vi "Facade.vi"(0 "Data In":T10=[{"Channel Name"=0, "Channel Alias"="", "Remove Channel"=FALSE, "Index"=0}], 2 "Display State In":T6={"Current Channels Info"=[], "Help Prefix"="", "Max Display Size"=8, "Max Size"=0, "Show Buttons"=TRUE, "Data Valid"=refnum, "Show Range"=FALSE, "Range Items"=[], "Range Index"=[]}, 3 "Container State":T9) -> (6 "Data Out":T10, 7 "Display State Out":T6={"Current Channels Info"=[], "Help Prefix"="", "Max Display Size"=8, "Max Size"=0, "Show Buttons"=TRUE, "Data Valid"=refnum, "Show Range"=FALSE, "Range Items"=[], "Range Index"=[]}, 8 "Action":T5)   [LabVIEW 2021, in "myRIO Channel List.xctl"]
uses:
  <vilib>/myRIO/Common/Express VI Framework/xctls/myRIO Channel List/myRIO Channel List.xctl
  <vilib>/myRIO/Common/Express VI Framework/xctls/myRIO Channel List/Data.ctl
  <vilib>/myRIO/Common/Express VI Framework/xctls/myRIO Channel List/typedefs/Channel Data.ctl
  <vilib>/myRIO/Common/Express VI Framework/xctls/myRIO Channel List/typedefs/Remove Channel.ctl
  <vilib>/_xctls/Container State.ctl
  <vilib>/myRIO/Common/Express VI Framework/xctls/myRIO Channel List/State.ctl
  <vilib>/myRIO/Common/Profile Manager Framework/typedefs/Channel Info.ctl
  <vilib>/myRIO/Common/Express VI Framework/typedefs/Data Validate Ref.ctl
  <vilib>/_xctls/Action.ctl
  <vilib>/myRIO/Common/Express VI Framework/xctls/myRIO Channel List/typedefs/Channel View.ctl
  <vilib>/myRIO/Common/Express VI Framework/xctls/myRIO Channel List/typedefs/Error Icon.ctl
  <vilib>/myRIO/Common/Express VI Framework/xctls/myRIO Channel List/typedefs/Add Channel.ctl
  <vilib>/myRIO/Common/Express VI Framework/xctls/myRIO Channel List/typedefs/Update State.ctl
  <vilib>/_xctls/XControlSupport.lvlib
panel:
  in  "Add Channel":T1
  in  "Channels":T2[](array[typedef])
  in  "Scrollbar":i32(c297)
  # "Channel:"
  # "Custom channel name:"
  # "Range:"
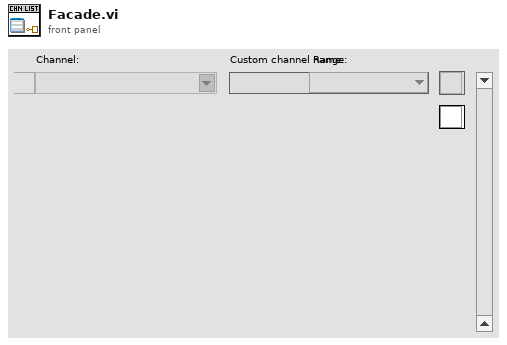
[diagram p1: front panel]
types:
  T1 = typedef "myRIO Channel List.xctl/Add Channel.ctl" = bool
  T2 = typedef "myRIO Channel List.xctl/Channel View.ctl" = cluster{"Error Icon":T3, "Channel Name":string, "Channel Alias":string, "Remove Channel":T4, "Index":i32, "Range":i32}
  T3 = typedef "myRIO Channel List.xctl/Error Icon.ctl" = bool
  T4 = typedef "myRIO Channel List.xctl/Remove Channel.ctl" = bool
  T5 = typedef "XControlSupport.lvlib/Action.ctl" = cluster{"Data Changed?":bool, "State Changed?":bool, "Action Name":string}
  T6 = typedef "myRIO Channel List.xctl/State.ctl" = cluster{"Current Channels Info":T7[], "Help Prefix":string, "Max Display Size":i32, "Max Size":i32, "Show Buttons":bool, "Data Valid":T8, "Show Range":bool, "Range Items":string[], "Range Index":i32[]}
  T7 = typedef "Channel Info.ctl" = cluster{"Channel Name":string, "Alias":string, "Used?":bool, "Not Support?":bool, "Property Bundle":cluster{"Name":string, "Value":variant}[]}
  T8 = typedef "Data Validate Ref.ctl" = refnum<user-event>
  T9 = typedef "XControlSupport.lvlib/Container State.ctl" = cluster{"Indicator?":bool, "Run Mode?":bool, " Refnum":refnum<vi>}
  T10 = typedef "myRIO Channel List.xctl/Data.ctl" = T11[]
  T11 = typedef "myRIO Channel List.xctl/Channel Data.ctl" = cluster{"Channel Name":u16, "Channel Alias":string, "Remove Channel":T4, "Index":i32}
  T12 = typedef "myRIO Channel List.xctl/Update State.ctl" = enum16{"Defer Update", "Allow Update", "Update Channel List", "Update Values", "Update Value", "Update Channel", "Update Index", "Update Scrollbar", "Update Buttons", "Update Container", "Update Help", "Show Or Hide Range"}
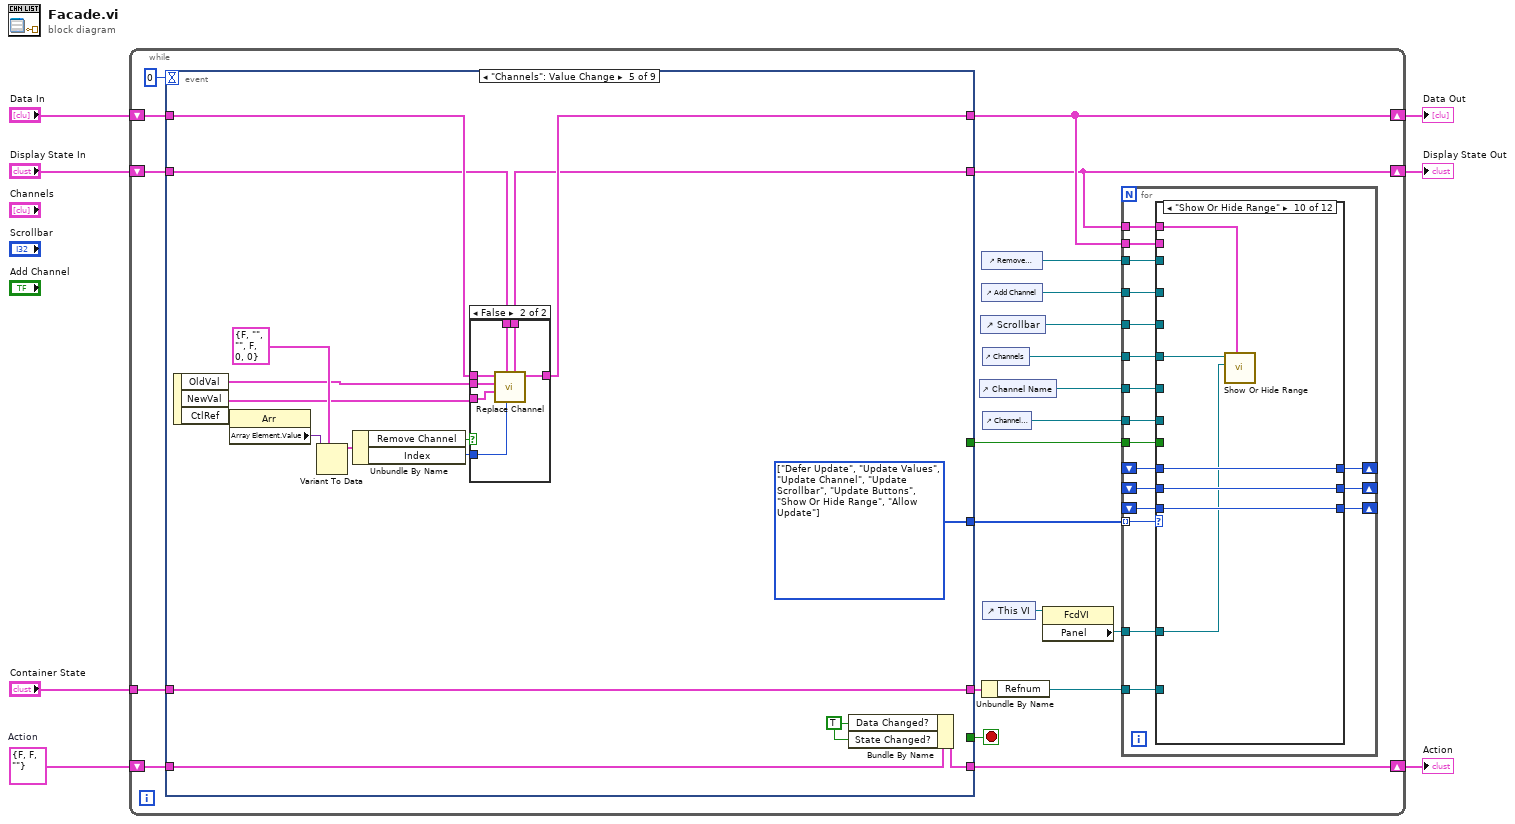
[diagram p0: block diagram]
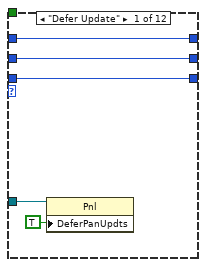
[diagram p2: hidden frame]
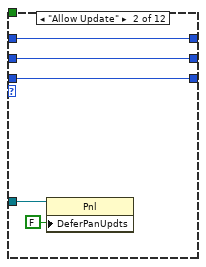
[diagram p3: hidden frame]
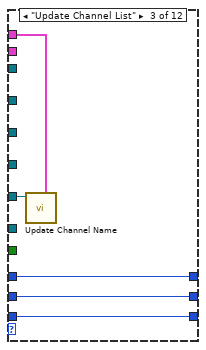
[diagram p4: hidden frame]
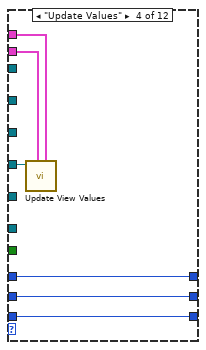
[diagram p5: hidden frame]
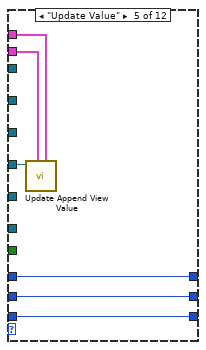
[diagram p6: hidden frame]
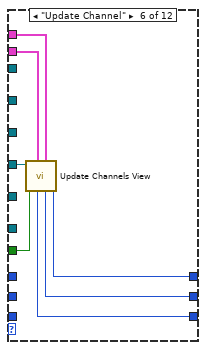
[diagram p7: hidden frame]
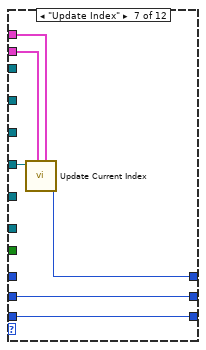
[diagram p8: hidden frame]
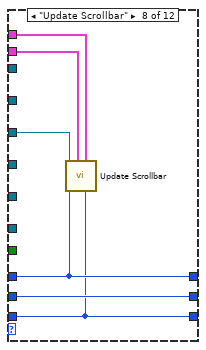
[diagram p9: hidden frame]
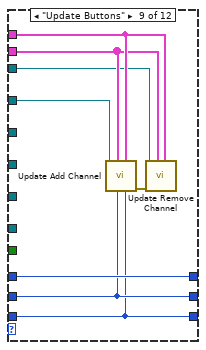
[diagram p10: hidden frame]
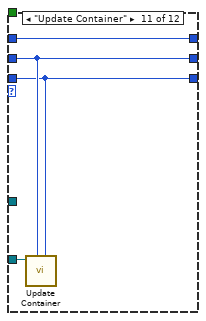
[diagram p11: hidden frame]
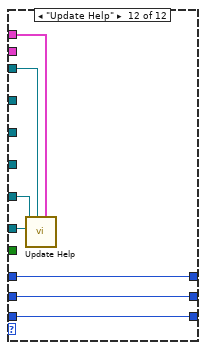
[diagram p12: hidden frame]
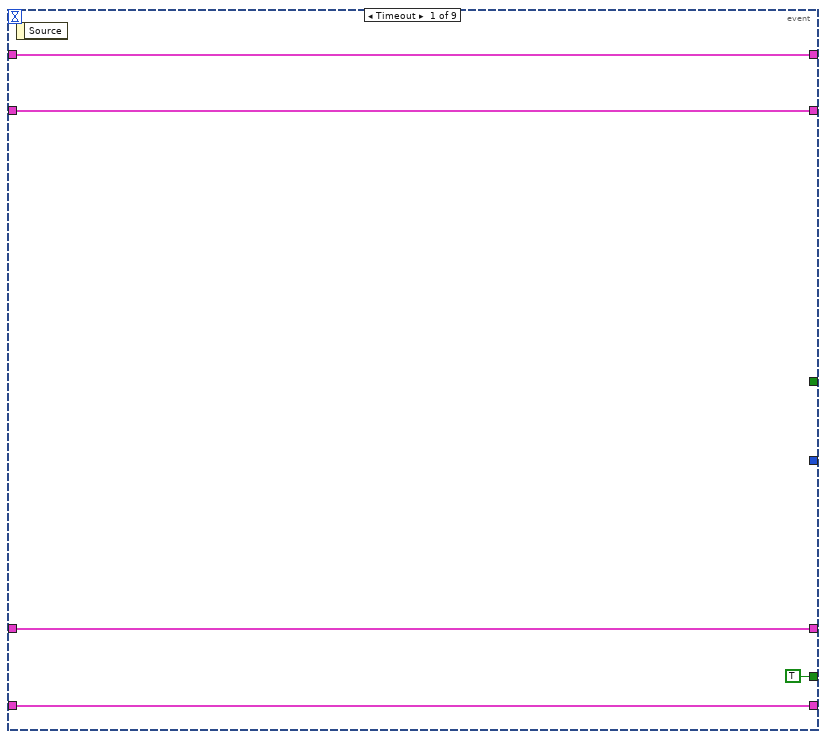
[diagram p13: hidden frame]
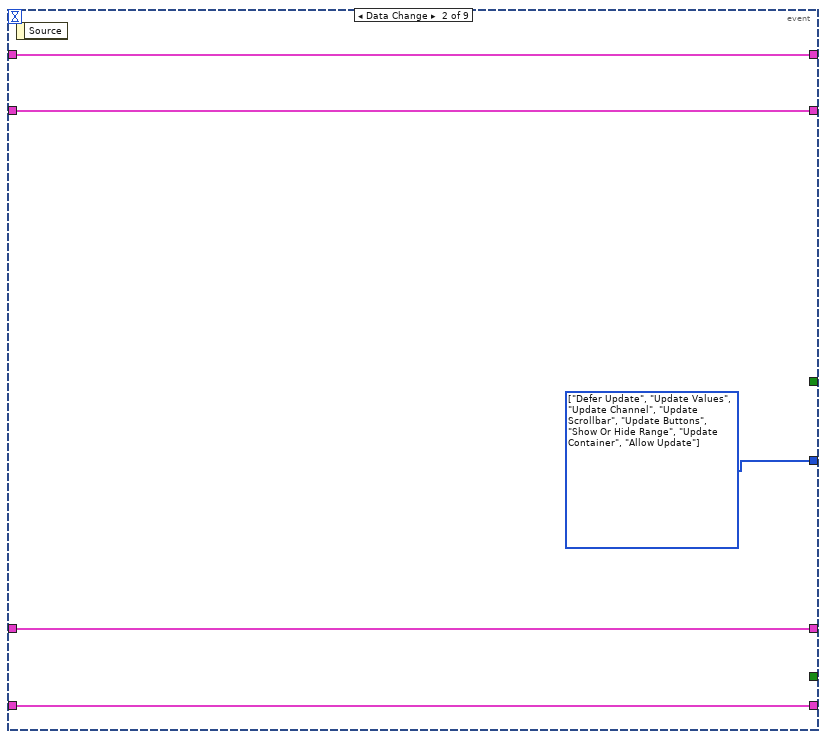
[diagram p14: hidden frame]
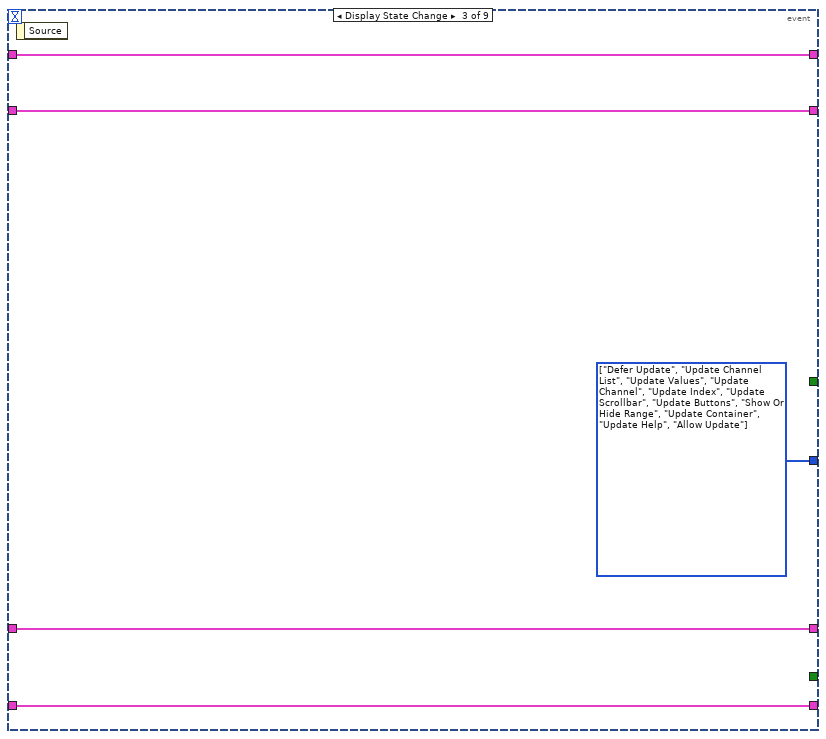
[diagram p15: hidden frame]
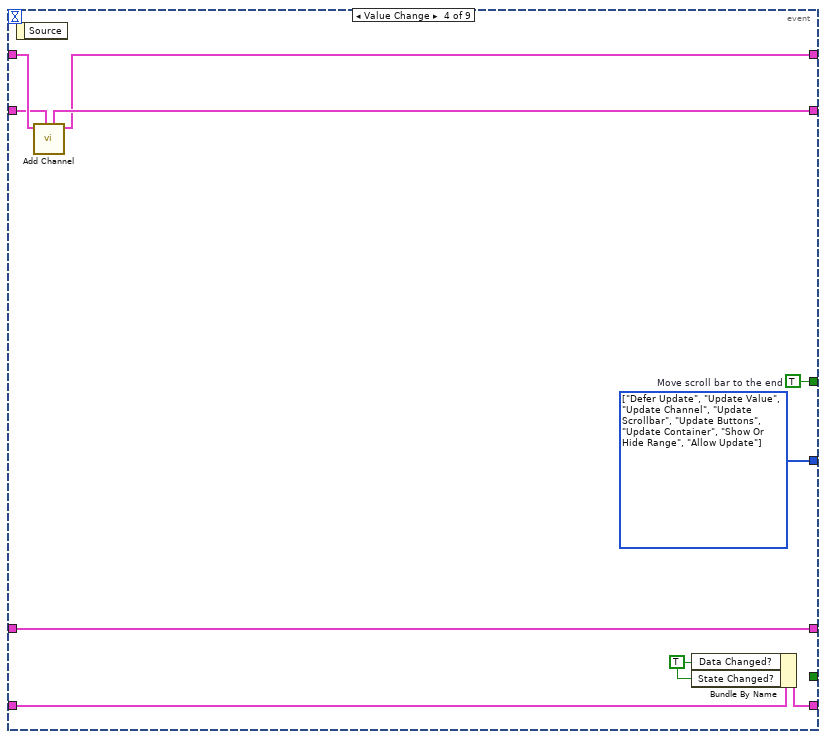
[diagram p16: hidden frame]
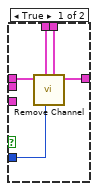
[diagram p17: hidden frame]
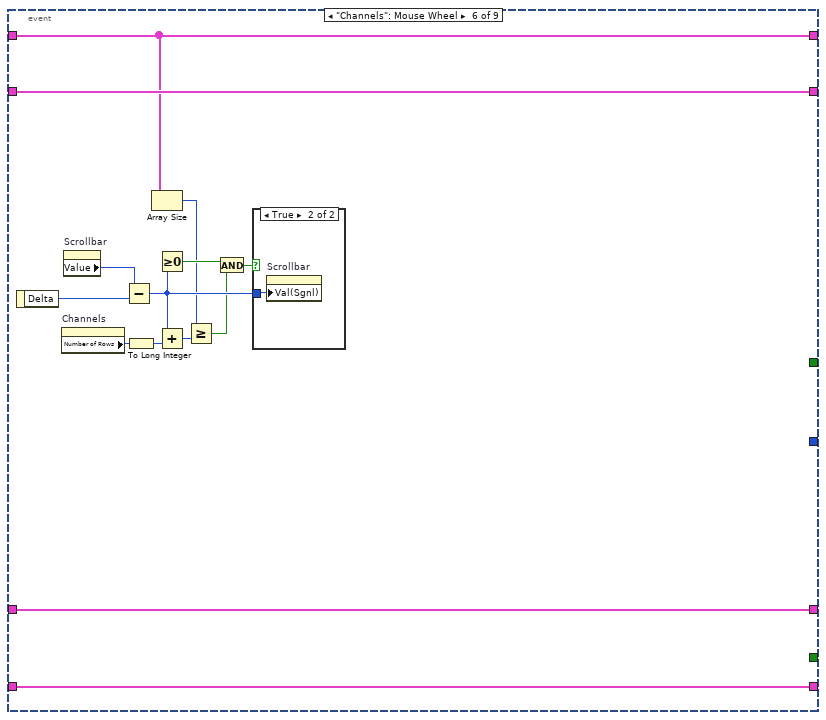
[diagram p18: hidden frame]
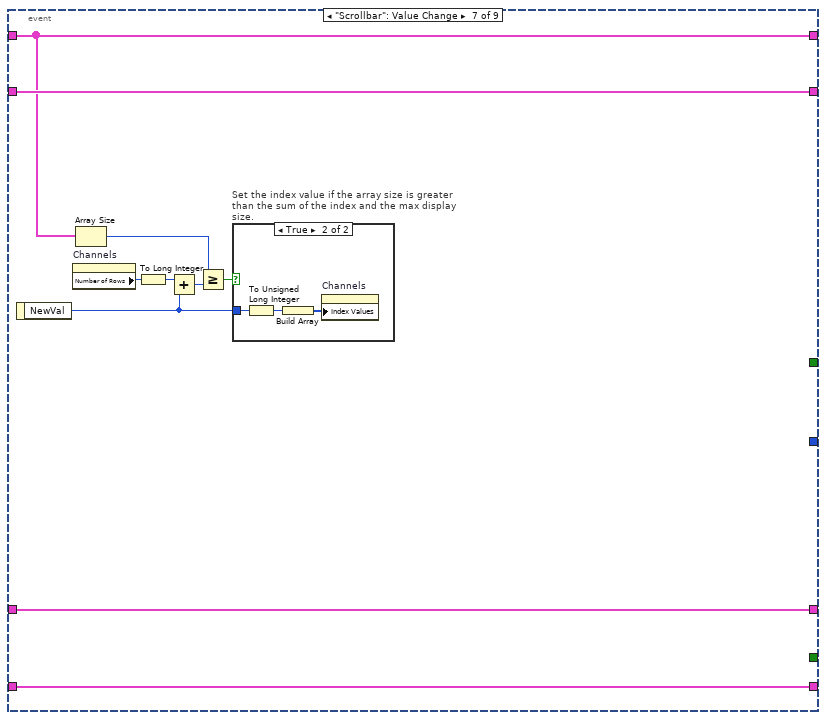
[diagram p20: hidden frame]
diagram:
  w3 = T5 {"Data Changed?"=FALSE, "State Changed?"=FALSE, "Action Name"=""}  # Action
  n1 = while {
    shift-right: [w20] -> w5
    shift-left: "Display State In" -> [w28]
    tunnel: "Container State" -> [w27]
    shift-right: [w21] -> w7
    shift-left: "Data In" -> [w26]
    shift-right: [w24] -> w4
    shift-left: w3 -> [w25]
    stop <- w23 stop-if-true
    n2 = event shown="[4] \"Channels\": Value Change" {
      selector: _ -> [_ _ _ _ _ _ _ _ _]
      dyn-events: _ -> [_ _ _ _ _ _ _ _ _]
      timeout: 0 -> [_ _ _ _ _ _ _ _ _]
      tunnel: w28 -> [w121 w126 w129 w139 w149 w185 w193 w203 w207]
      tunnel: [w121 w126 w129 w138 w148 w185 w193 w203 w207] -> w20
      tunnel: [TRUE _ _ _ _ _ _ _ _] -> w23
      tunnel: w27 -> [w118 w124 w130 w137 w152 w177 w187 w200 w204]
      tunnel: w26 -> [w120 w125 w131 w141 w154 w172 w191 w202 w206]
      tunnel: [w120 w125 w131 w136 w153 w172 w191 w202 w206] -> w21
      tunnel: [w122 w127 w132 w140 w151 w184 w196 w201 w205] -> w24
      tunnel: w25 -> [w122 w127 w132 w142 w159 w184 w196 w201 w205]
      tunnel: [_ w123 w128 w133 w143 _ _ _ _] -> w22
      tunnel: [w118 w124 w130 w137 w152 w177 w187 w200 w204] -> w14
      tunnel: [_ _ _ w134 _ _ _ _ _] -> w8
      event Timeout {
        n3 = event-data() -> ()  [unwired: 1 in, 1 out]
      }
      event Data Change {
        w123 = T12[] [enum."Defer Update", enum."Update Values", enum."Update Channel", enum."Update Scrollbar", enum."Update Buttons", enum."Show Or Hide Range", enum."Update Container", enum."Allow Update"] items=["Defer Update", "Allow Update", "Update Channel List", "Update Values", "Update Value", "Update Channel", "Update Index", "Update Scrollbar", "Update Buttons", "Update Container", "Update Help", "Show Or Hide Range"]
        n4 = event-data() -> ()  [unwired: 1 in, 1 out]
      }
      event Display State Change {
        w128 = T12[] [enum."Defer Update", enum."Update Channel List", enum."Update Values", enum."Update Channel", enum."Update Index", enum."Update Scrollbar", enum."Update Buttons", enum."Show Or Hide Range", enum."Update Container", enum."Update Help", enum."Allow Update"] items=["Defer Update", "Allow Update", "Update Channel List", "Update Values", "Update Value", "Update Channel", "Update Index", "Update Scrollbar", "Update Buttons", "Update Container", "Update Help", "Show Or Hide Range"]
        n5 = event-data() -> ()  [unwired: 1 in, 1 out]
      }
      event Value Change {
        w133 = T12[] [enum."Defer Update", enum."Update Value", enum."Update Channel", enum."Update Scrollbar", enum."Update Buttons", enum."Update Container", enum."Show Or Hide Range", enum."Allow Update"] items=["Defer Update", "Allow Update", "Update Channel List", "Update Values", "Update Value", "Update Channel", "Update Index", "Update Scrollbar", "Update Buttons", "Update Container", "Update Help", "Show Or Hide Range"]
        w134 = TRUE  # Move scroll bar to the end
        w135 = TRUE ("Data Changed?")
        n6 = event-data() -> ()  [unwired: 1 in, 1 out]
        n7 = call <vilib>:"Add Channel.vi"("Display State In"=w139, "Channels In"=w141) -> ("Channels Out"=w136:T10, "Display State Out"=w138:T6)  [unwired: 8 in]
        n8 = Bundle By Name(cluster=w142, "Data Changed?"=w135, "State Changed?"=w135) -> (w140:T5)
      }
      event "Channels": Value Change {
        w143 = T12[] [enum."Defer Update", enum."Update Values", enum."Update Channel", enum."Update Scrollbar", enum."Update Buttons", enum."Show Or Hide Range", enum."Allow Update"] items=["Defer Update", "Allow Update", "Update Channel List", "Update Values", "Update Value", "Update Channel", "Update Index", "Update Scrollbar", "Update Buttons", "Update Container", "Update Help", "Show Or Hide Range"]
        w144 = TRUE ("Data Changed?")
        n9 = event-data() -> ("OldVal"=w147:T2[], "NewVal"=w150:T2[], "CtlRef"=w158:refnum<vi>)  [unwired: 1 in]
        n10 = property class="Arr"(reference=w158) -> ("Array Element.Value"=w157:variant)  [unwired: 1 in, 2 out]
        n11 = Variant To Data(type=T2 {"Error Icon"=FALSE, "Channel Name"="", "Channel Alias"="", "Remove Channel"=FALSE, "Index"=0, "Range"=0} ("Channel"), Variant=w157) -> (data=w155:T2)  [unwired: 1 in, 1 out]
        n12 = Unbundle By Name(w155) -> ("Remove Channel"=w146:T4, "Index"=w145:i32)
        n13 = case shown="False" w146 {
          tunnel: w145 -> [w160 w165]
          tunnel: w154 -> [w164 w171]
          tunnel: [w163 w170] -> w153
          tunnel: w149 -> [w162 w169]
          tunnel: [w161 w168] -> w148
          tunnel: w150 -> [_ w166]
          tunnel: w147 -> [_ w167]
          frame True {
            n14 = call <vilib>:"Remove Channel.vi"("Index"=w160, "Display State In"=w162, "Channels In"=w164) -> ("Channels Out"=w163:T10, "Display State Out"=w161:T6)  [unwired: 7 in]
          }
          frame False {
            n15 = call <vilib>:"Replace Channel.vi"("Index"=w165, "Display State In"=w169, "New Channels View"=w166, "Old Channels View"=w167, "Channels In"=w171) -> ("Channels Out"=w170:T10, "Display State Out"=w168:T6)  [unwired: 4 in, 1 out]
          }
        }
        n16 = Bundle By Name(cluster=w159, "Data Changed?"=w144, "State Changed?"=w144) -> (w151:T5)
      }
      event "Channels": Mouse Wheel {
        n17 = event-data() -> ("Delta"=w179:i32)  [unwired: 1 in]
        n18 = property on="Channels" class="Arr"() -> ("Number of Rows"=w178:u32)  [unwired: 2 in, 2 out]
        n19 = property on="Scrollbar" class="Scroll (strict)"() -> ("Value"=w176:i32)  [unwired: 2 in, 2 out]
        n20 = Subtract(x=w176, y=w179) -> (x-y=w182:i32)
        n21 = To Long Integer(number=w178) -> (32bit integer=w175:i32)
        n22 = Array Size(array=w172) -> (size(s)=w174:i32)
        n23 = Greater Or Equal To 0?(x=w182) -> (x >= 0?=w181:bool)
        n24 = Add(x=w182, y=w175) -> (x+y=w183:i32)
        n25 = Greater Or Equal?(x=w174, y=w183) -> (x >= y?=w173:bool)
        n26 = And(x=w181, y=w173) -> (x .and. y?=w180:bool)
        n27 = case shown="True" w180 {
          tunnel: w182 -> [_ w186]
          frame False {
          }
          frame True {
            n28 = property on="Scrollbar" class="Scroll (strict)"("Val(Sgnl)"=w186) -> ()  [unwired: 2 in, 2 out]
          }
        }
      }
      event "Scrollbar": Value Change {
        n29 = event-data() -> ("NewVal"=w189:i32)  [unwired: 1 in]
        n30 = property on="Channels" class="Arr"() -> ("Number of Rows"=w192:u32)  [unwired: 2 in, 2 out]
        n31 = Array Size(array=w191) -> (size(s)=w188:i32)
        n32 = To Long Integer(number=w192) -> (32bit integer=w190:i32)
        n33 = Add(x=w190, y=w189) -> (x+y=w195:i32)
        n34 = Greater Or Equal?(x=w188, y=w195) -> (x >= y?=w194:bool)
        n35 = case "Set the index value if the array size is greater than the sum of the index and the max display size." shown="True" w194 {
          tunnel: w189 -> [_ w199]
          frame False {
          }
          frame True {
            n36 = To Unsigned Long Integer(number=w199) -> (unsigned 32bit integer=w197:u32)
            n37 = Build Array(w197) -> (w198:u32[])
            n38 = property on="Channels" class="Arr"("Index Values"=w198) -> ()  [unwired: 2 in, 2 out]
          }
        }
      }
      event Direction Change {
        n39 = event-data() -> ()  [unwired: 1 in, 4 out]
      }
      event Exec State Change {
        n40 = event-data() -> ()  [unwired: 1 in, 4 out]
      }
    }
    n41 = control-ref of="Channel Name"() -> (w15:refnum<vi>)
    n42 = control-ref of="Scrollbar"() -> (w17:refnum<vi>)
    n43 = control-ref of="Remove Channel"() -> (w19:refnum<vi>)
    n44 = control-ref of="Add Channel"() -> (w18:refnum<vi>)
    n45 = Unbundle By Name(w14) -> ("Refnum"=w13:refnum<vi>)
    n46 = control-ref of="Channels"() -> (w16:refnum<vi>)
    n47 = control-ref of="Channel Alias"() -> (w9:refnum<vi>)
    n48 = control-ref of="This VI"() -> (w12:refnum<vi>)
    n49 = property class="FcdVI"(reference=w12) -> ("Panel"=w11:refnum<vi>)  [unwired: 1 in, 2 out]
    n50 = for {
      tunnel: w22 -> [w46] mode=indexing
      tunnel: w19 -> [w45]
      tunnel: w18 -> [w44]
      tunnel: w17 -> [w43]
      tunnel: w21 -> [w42]
      tunnel: w20 -> [w41]
      tunnel: w15 -> [w40]
      tunnel: w16 -> [w39]
      shift-right: [w38] -> _
      shift-left: _ -> [w37]
      shift-right: [w36] -> _
      shift-left: _ -> [w35]
      tunnel: w13 -> [w34]
      tunnel: w11 -> [w33]
      tunnel: w9 -> [w32]
      tunnel: w8 -> [w31]
      shift-right: [w30] -> _
      shift-left: _ -> [w29]
      n51 = case shown="\"Show Or Hide Range\"" w46 {
        tunnel: w45 -> [_ _ _ _ _ _ _ _ w97 _ _ w113]
        tunnel: w44 -> [_ _ _ _ _ _ _ _ w96 _ _ _]
        tunnel: w43 -> [_ _ _ _ _ _ _ w90 _ _ _ _]
        tunnel: w42 -> [_ _ _ w63 w69 w78 w84 w91 w98 _ _ _]
        tunnel: w41 -> [_ _ w60 w67 w73 w79 w85 w92 w99 w103 _ w112]
        tunnel: w40 -> [_ _ w61 _ _ _ _ _ _ _ _ w114]
        tunnel: w39 -> [_ _ _ w64 w70 w80 w86 _ _ w102 _ _]
        tunnel: [w50 w55 w59 w66 w72 w75 w83 w89 w94 w106 w108 w116] -> w38
        tunnel: w37 -> [w50 w55 w59 w66 w72 _ w83 w89 w94 w106 w108 w116]
        tunnel: [w51 w56 w58 w65 w71 w74 w82 w87 w93 w105 w107 w117] -> w36
        tunnel: w35 -> [w51 w56 w58 w65 w71 _ w82 w87 w93 w105 w107 w117]
        tunnel: w34 -> [_ _ _ _ _ _ _ _ _ _ w110 _]
        tunnel: w33 -> [w49 w54 _ _ _ _ _ _ _ w101 _ _]
        tunnel: w32 -> [_ _ _ _ _ _ _ _ _ _ _ w115]
        tunnel: w31 -> [_ _ _ _ _ w77 _ _ _ _ _ _]
        tunnel: [w47 w52 w57 w62 w68 w76 w81 w88 w95 w104 w109 w111] -> w30
        tunnel: w29 -> [w47 w52 w57 w62 w68 _ _ w88 w95 w104 w109 w111]
        frame "Defer Update" {
          n52 = property class="Pnl"(reference=w49, "DeferPanUpdts"=TRUE ("Defer Panel Updates")) -> ()  [unwired: 1 in, 2 out]
        }
        frame "Allow Update" {
          n53 = property class="Pnl"(reference=w54, "DeferPanUpdts"=FALSE ("Defer Panel Updates")) -> ()  [unwired: 1 in, 2 out]
        }
        frame "Update Channel List" {
          n54 = call <vilib>:"Update Channel Name.vi"("Display State In"=w60, "Channel Name Reference"=w61) -> ()  [unwired: 9 in, 1 out]
        }
        frame "Update Values" {
          n55 = call <vilib>:"Update View Values.vi"("Display State In"=w67, "Channels In"=w63, "Channels Reference"=w64) -> ()  [unwired: 9 in]
        }
        frame "Update Value" {
          n56 = call <vilib>:"Update Append View Value.vi"("Display State In"=w73, "Channels In"=w69, "Channels Reference"=w70) -> ()  [unwired: 9 in]
        }
        frame "Update Channel" {
          n57 = call <vilib>:"Update Channels View.vi"("Display State In"=w79, "Channels In"=w78, "Move Scorllbar to End"=w77, "Channels Reference"=w80) -> ("Current Index"=w76:i32, "Number of Row"=w75:i32, "Area Height"=w74:u32)  [unwired: 4 in, 1 out]
        }
        frame "Update Index" {
          n58 = call <vilib>:"Update Current Index.vi"("Display State In"=w85, "Channels In"=w84, "Channels Reference"=w86) -> ("Current Index"=w81:i32)  [unwired: 7 in, 1 out]
        }
        frame "Update Scrollbar" {
          n59 = call <vilib>:"Update Scrollbar.vi"("Area Height"=w87, "Display State In"=w92, "Channels In"=w91, "Current Index"=w88, "Scrollbar Reference"=w90) -> ()  [unwired: 6 in, 1 out]
        }
        frame "Update Buttons" {
          n60 = call <vilib>:"Update Add Channel.vi"("Area Height"=w93, "Display State In"=w99, "Number of Row"=w94, "Channels In"=w98, "Add Channel Reference"=w96) -> ("error out"=w100:errorcluster)  [unwired: 6 in]
          n61 = call <vilib>:"Update Remove Channel.vi"("Display State In"=w99, "Channels In"=w98, "error in (no error)"=w100, "Remove Channel Reference"=w97) -> ()  [unwired: 7 in, 1 out]
        }
        frame "Show Or Hide Range" {
          n62 = call <vilib>:"Show Or Hide Range.vi"("Display State In"=w103, "Panel"=w101, "Channels Reference"=w102) -> ()  [unwired: 8 in, 1 out]
        }
        frame "Update Container" {
          n63 = call <vilib>:"Update Container.vi"("Area Height"=w107, "Number of Row"=w108, "Container Reference"=w110) -> ()  [unwired: 8 in, 1 out]
        }
        frame "Update Help" {
          n64 = call <vilib>:"Update Help.vi"("Display State In"=w112, "Remove Channel"=w113, "Channel Alias"=w115, "Channel Name"=w114) -> ()  [unwired: 8 in]
        }
      }
    }
  }
  "Display State Out" <- w5
  "Data Out" <- w7
  "Action" <- w4
